vi "2086发送2.vi"() -> ()   [LabVIEW 2016, in "数据传输系统-06.lvlib"]
uses:
  <vilib>/Utility/config.llb/Write Key (String).vi
  <vilib>/Utility/config.llb/Read Key (String).vi
  <vilib>/Utility/config.llb/NI_LVConfig.lvlib
panel:
  out "数据发送起始时间":timestamp format="%<%.3X\n%Y/%m/%d>T"
  out "数据拆分":bool
  in  "设备类型":string(combo)="010200"
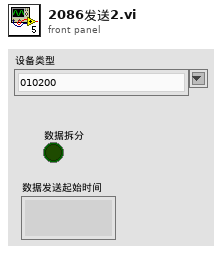
[diagram p1: front panel]
types:
  T1 = cluster{"CODMn":string, "CODCr":string, "DO":string, "铜":string, "PH":string, "氨氮":string, "比电导率":string, "水温":string, "COD":string, "浊度":string, "总氮":string, "总磷":string, "叶绿素a":string, "藻密度":string, "水位":string, "流速":string, "方向":string, "瞬时流量":string, "累积流量":string, "正累积流量":string, "负累积流量":string, "亚硝酸盐":string, "硫化物":string, "ORP":string, "铅":string, "镉":string, "锌":string, "镍":string, "锰":string, "汞":string, "气温":string, "气压":string, "风速":string, "风向":string, "空气温度":string, "相对湿度":string, "分钟雨量":string, "小时雨量":string, "日雨量":string, "累积雨量":string, "盐度":string, "磷酸盐":string, "硝氮":string, "氟化物":string, "挥发酚":string, "氯化物":string, "蓝绿藻":string, "余氯":string, "综合生物毒性":string, "艏向":string, "横摇":string, "纵摇":string, "分层标志":string, "层状态1":string, "层状态2":string, "水平平均流速":string, "流向":string, "北向流速分量":string, "东向流速分量":string, "垂直流速分量":string, "最大波高":string, "最大波周期":string, "1/10波高":string, "1/10波周期":string, "有效波高":string, "有效波周期":string, "平均波高":string, "平均波周期":string, "波向":string, "波个数":string, "水深":string, "X轴流速":string, "Y轴流速":string, "信号强度":string, "电压":string, "悬浮物":string}
  T2 = cluster{"QN":string, "ST":string, "CN":string, "PW":string, "MN":string, "FLAG":string, "PNUM":string, "PNO":string, "CP":string}
  T3 = typedef "LVComboBoxStrsAndValuesArrayTypeDef.ctl" = cluster{"String":string, "Value":string}[]
  T4 = typedef "数据传输系统-06.lvlib/应用环境.ctl" = enum16{"STD", "GB212", "婉仪平台"}
  T5 = cluster{"setini":string, "sysini":string, "hechaini":string, "actualwrite":string, "actualread":string, "datasent":string, "反控命令信息队列":string, "反控与仪器交互":string}
  T6 = cluster{"time1":string, "time2":string, "time3":string, "time4":string, "time5":string, "time6":string, "time7":string, "time8":string, "time9":string, "time10":string, "time11":string, "time12":string, "time13":string, "time14":string, "time15":string, "time16":string, "time17":string, "time18":string, "time19":string, "time20":string, "time21":string, "time22":string, "time23":string, "time24":string, "time25":string, "time26":string, "time27":string, "time28":string, "time29":string, "time30":string, "time31":string, "time32":string, "time33":string, "time34":string, "time35":string, "time36":string, "time37":string, "time38":string, "time39":string, "time40":string, "time41":string, "time42":string, "time43":string, "time44":string, "time45":string, "time46":string, "time47":string, "time48":string, "time49":string, "time50":string, "time51":string, "time52":string, "time53":string, "time54":string, "time55":string, "time56":string, "time57":string, "time58":string, "time59":string, "time60":string, "time61":string, "time62":string, "time63":string, "time64":string, "time65":string, "time66":string, "time67":string, "time68":string, "time69":string, "time70":string, "time71":string, "time72":string, "time73":string, "time74":string, "time75":string, "time76":string}
  T7 = cluster{"水样数据索引[0]":string, "水样数据索引[1]":string, "水样数据索引[2]":string, "水样数据索引[3]":string, "水样数据索引[4]":string, "水样数据索引[5]":string, "水样数据索引[6]":string, "水样数据索引[7]":string, "水样数据索引[8]":string, "水样数据索引[9]":string, "水样数据索引[10]":string, "水样数据索引[11]":string, "水样数据索引[12]":string, "水样数据索引[13]":string, "水样数据索引[14]":string, "水样数据索引[15]":string, "水样数据索引[16]":string, "水样数据索引[17]":string, "水样数据索引[18]":string, "水样数据索引[19]":string, "水样数据索引[20]":string, "水样数据索引[21]":string, "水样数据索引[22]":string, "水样数据索引[23]":string, "水样数据索引[24]":string, "水样数据索引[25]":string, "水样数据索引[26]":string, "水样数据索引[27]":string, "水样数据索引[28]":string, "水样数据索引[29]":string, "水样数据索引[30]":string, "水样数据索引[31]":string, "水样数据索引[32]":string, "水样数据索引[33]":string, "水样数据索引[34]":string, "水样数据索引[35]":string, "水样数据索引[36]":string, "水样数据索引[37]":string, "水样数据索引[38]":string, "水样数据索引[39]":string, "水样数据索引[40]":string, "水样数据索引[41]":string, "水样数据索引[42]":string, "水样数据索引[43]":string, "水样数据索引[44]":string, "水样数据索引[45]":string, "水样数据索引[46]":string, "水样数据索引[47]":string, "水样数据索引[48]":string, "水样数据索引[49]":string, "水样数据索引[50]":string, "水样数据索引[51]":string, "水样数据索引[52]":string, "水样数据索引[53]":string, "水样数据索引[54]":string, "水样数据索引[55]":string, "水样数据索引[56]":string, "水样数据索引[57]":string, "水样数据索引[58]":string, "水样数据索引[59]":string, "水样数据索引[60]":string, "水样数据索引[61]":string, "水样数据索引[62]":string, "水样数据索引[63]":string, "水样数据索引[64]":string, "水样数据索引[65]":string, "水样数据索引[66]":string, "水样数据索引[67]":string, "水样数据索引[68]":string, "水样数据索引[69]":string, "水样数据索引[70]":string, "水样数据索引[71]":string, "水样数据索引[72]":string, "水样数据索引[73]":string, "水样数据索引[74]":string, "水样数据索引[75]":string}
  T8 = typedef "NI_LVConfig.lvlib/Config Data RefNum.ctl" = refnum<k1>
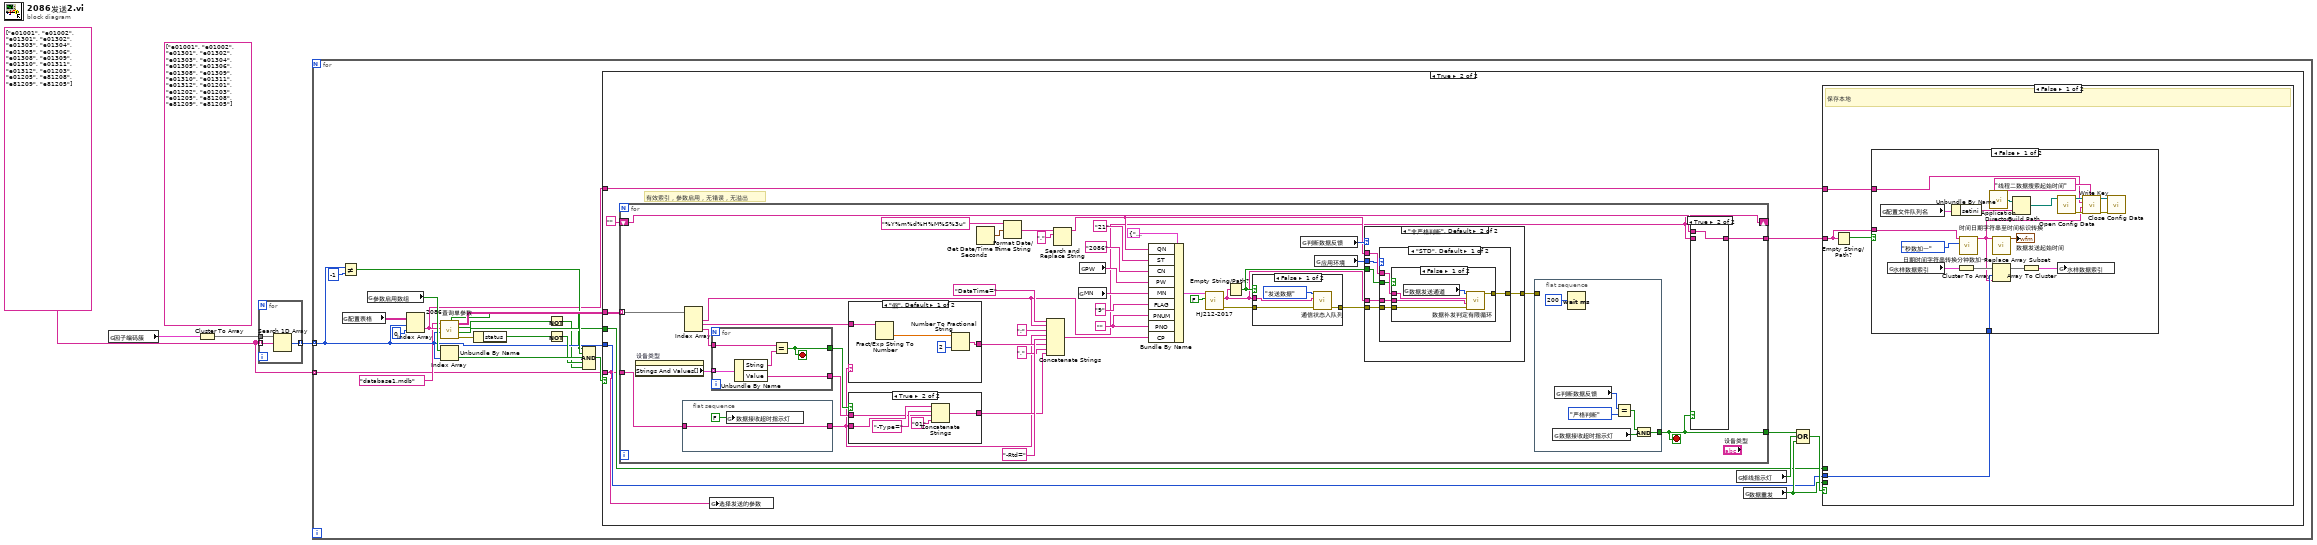
[diagram p0: block diagram]
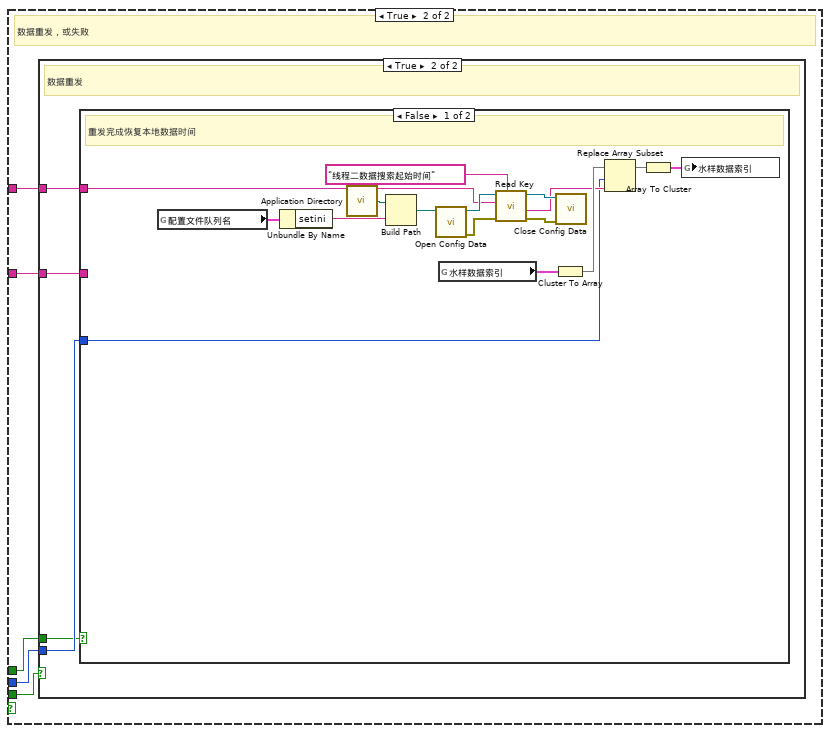
[diagram p4: hidden frame]
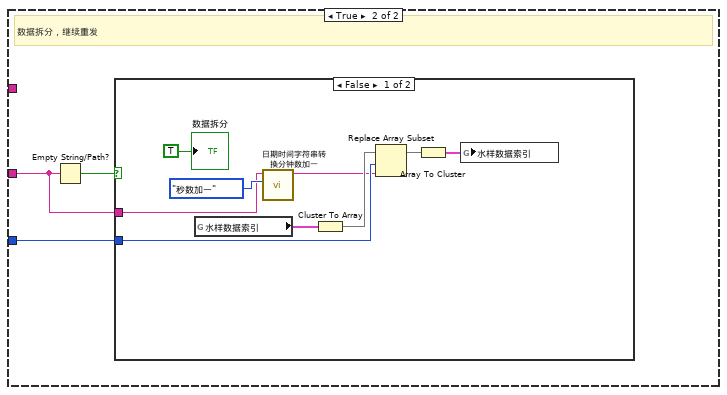
[diagram p6: hidden frame]
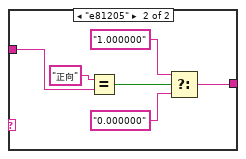
[diagram p9: hidden frame]
diagram:
  w1 = string[] ["e01001", "e01002", "e01301", "e01302", "e01303", "e01304", "e01305", "e01306", "e01308", "e01309", "e01310", "e01311", "e01312", "e01203", "e01205", "e81208", "e81209", "e81205"]
  (unwired) string[] ["e01001", "e01002", "e01301", "e01302", "e01303", "e01304", "e01305", "e01306", "e01308", "e01309", "e01310", "e01311", "e01312", "e01201", "e01202", "e01203", "e01205", "e81208", "e81209", "e81205"]
  n1 = global read "断电保存全局.vi" "因子编码簇"() -> (w4:T1)
  n2 = Cluster To Array(cluster=w4) -> (array=w3:string[])
  n3 = for {
    tunnel: w3 -> [w7]
    tunnel: w1 -> [w6] mode=indexing
    tunnel: [w5] -> w2 mode=indexing
    n4 = Search 1D Array(1D array=w7, element=w6) -> (index of element=w5:i32)  [unwired: 1 in]
  }
  n5 = for {
    tunnel: w2 -> [w11] mode=indexing
    tunnel: w1 -> [w10] mode=indexing
    n6 = Not Equal?(x=w11, y=-1) -> (x != y?=w21:bool)
    n7 = global read "断电保存全局.vi" "配置表格"() -> (w25:string[][])
    n8 = global read "断电保存全局.vi" "参数启用数组"() -> (w22:bool[])
    n9 = Index Array(array=w25, index (row)=w11, index (col)=0 ("y")) -> (element=w19:string)
    n10 = call "2086查询单参数.vi"("索引"=w11, "table"=w19, "database"="database1.mdb") -> ("error out"=w16:errorcluster, "拆分数据"=w17:bool, "database溢出"=w12:bool, "data"=w23:string[][], "有数据"=w8:bool)  [unwired: 4 in]
    n11 = Index Array(array=w22, index=w11) -> (element=w20:bool)
    n12 = Unbundle By Name(w16) -> ("status"=w15:bool)
    n13 = Not(x=w12) -> (.not. x?=w9:bool)
    n14 = Not(x=w15) -> (.not. x?=w14:bool)
    n15 = Compound Arithmetic op=AND ("复合运算")(w8, w21, w20, w14, w9) -> (w13:bool)
    n16 = case shown="True" w13 {
      tunnel: w23 -> [_ w37]
      tunnel: w10 -> [_ w27]
      tunnel: w19 -> [_ w32]
      tunnel: w11 -> [_ w31]
      tunnel: w17 -> [_ w30]
      frame False {
      }
      frame True {
        # "有效索引，参数启用，无错误，无溢出"
        n17 = for {
          tunnel: w37 -> [w106] mode=indexing
          tunnel: w27 -> [w98]
          tunnel: [w103] -> w36
          shift-right: [w101] -> _
          shift-left: "" -> [w102]
          tunnel: [w100] -> w29
          stop <- w103 stop-if-true
          w127 = ""
          n18 = property on="设备类型" class="CmbBox"() -> ("Strings And Values[]"=w120:T3)  [unwired: 2 in, 2 out]
          n19 = flat-sequence {
            tunnel: [w139] -> w99
            tunnel: w98 -> [w139]
            frame #0 {
              n20 = global write "全局 数据发送重叠.vi" "数据接收超时指示灯"(FALSE ("数据接收超时指示灯")) -> ()
            }
          }
          n21 = Index Array(array=w106) -> (element #1=w101:string, element #2=w105:string, element #3=w117:string)  [unwired: 3 in]
          n22 = for {
            tunnel: w120 -> [w188] mode=indexing
            tunnel: w117 -> [w186]
            tunnel: [w185] -> w118
            tunnel: [w184] -> w119
            stop <- w184 stop-if-true
            n23 = Unbundle By Name(w188) -> ("String"=w187:string, "Value"=w185:string)
            n24 = Equal?(x=w186, y=w187) -> (x = y?=w184:bool)
          }
          n25 = case shown="\"假\", Default" w99 {
            tunnel: w105 -> [w143 w151]
            tunnel: [w142 w146] -> w104
            frame "假", Default {
              n26 = Fract/Exp String To Number(string=w143) -> (number=w145:dbl)  [unwired: 3 in, 1 out]
              n27 = Number To Fractional String(number=w145, precision (6)=i16 2 ("精度(6)")) -> (F-format string=w142:string)  [unwired: 2 in]
            }
            frame "e81205" {
              n28 = Equal?(x="正向", y=w151) -> (x = y?=w149:bool)
              n29 = Select(t="1.000000" ("x"), s=w149, f="0.000000" ("x")) -> (s? t:f=w146:string)
            }
          }
          n30 = case shown="True" w119 {
            tunnel: w118 -> [_ w181]
            tunnel: w99 -> [_ w183]
            tunnel: [_ w179] -> w115
            frame False {
            }
            frame True {
              n31 = Concatenate Strings(w183, "-Type=" ("格式字符串"), w181, "01" ("字符串")) -> (w179:string)
            }
          }
          n32 = Get Date/Time In Seconds() -> (seconds since 1Jan1904=w135:timestamp)
          n33 = Format Date/Time String(time format string (%c)="%Y%m%d%H%M%S%3u" ("时间格式字符串(%c)"), seconds (now)=w135) -> (date/time string=w134:string)  [unwired: 1 in]
          n34 = Concatenate Strings("DataTime=" ("时间格式字符串(%c)"), w101, ";" ("字符串"), w99, "-Rtd=" ("时间格式字符串(%c)"), w104, "," ("字符串"), w115) -> (w125:string)
          n35 = Search and Replace String(input string=w134, search string="." ("搜索字符串")) -> (result string=w108:string)  [unwired: 6 in, 3 out]
          n36 = global read "断电保存全局.vi" "MN"() -> (w132:string)
          n37 = global read "断电保存全局.vi" "PW"() -> (w131:string)
          n38 = Bundle By Name(cluster=T2 {"QN"="", "ST"="", "CN"="", "PW"="", "MN"="", "FLAG"="", "PNUM"="", "PNO"="", "CP"=""} ("数据块"), "QN"=w108, "ST"="21", "CN"="2086", "PW"=w131, "MN"=w132, "FLAG"="9", "PNUM"=w127, "PNO"=w127, "CP"=w125) -> (w121:T2)
          n39 = call "HJ212-2017.vi"("PWD？"=FALSE, "数据段"=w121) -> ("error out"=w109:errorcluster, "通讯包字符串"=w110:string)  [unwired: 7 in, 1 out]
          n40 = Empty String/Path?(string/path=w110) -> (empty?=w114:bool)
          n41 = case shown="False" w114 {
            tunnel: [w161 w162] -> w112
            tunnel: w109 -> [w160 w162]
            tunnel: w110 -> [w158 _]
            frame False {
              n42 = call "通信状态入队列.vi"("错误输入（无错误）"=w160, "发送报文"=w158, "枚举"=enum16{"打开连接", "发送数据", "读取数据", "数据处理", "关闭连接"}."发送数据") -> ("错误输出"=w161:errorcluster)  [unwired: 8 in]
            }
            frame True {
            }
          }
          n43 = global read "断电保存全局.vi" "判断数据反馈"() -> (w111:enum16{"非严格判断", "严格判断", "不判断"})
          n44 = global read "断电保存全局.vi" "应用环境"() -> (w113:T4)
          n45 = case shown="\"非严格判断\", Default" w111 {
            tunnel: w110 -> [_ w168]
            tunnel: w112 -> [_ w167]
            tunnel: w108 -> [_ w166]
            tunnel: w113 -> [_ w165]
            tunnel: w114 -> [_ w164]
            tunnel: [_ w163] -> w107
            frame "不判断" {
            }
            frame "非严格判断", Default {
              n46 = case shown="\"STD\", Default" w165 {
                tunnel: w168 -> [w171 _]
                tunnel: w167 -> [w173 _]
                tunnel: w166 -> [w172 _]
                tunnel: w164 -> [w170 _]
                tunnel: [w169 _] -> w163
                frame "STD", Default {
                  n47 = case shown="False" w170 {
                    tunnel: w173 -> [w178 _]
                    tunnel: w172 -> [w176 _]
                    tunnel: w171 -> [w175 _]
                    tunnel: [w174 _] -> w169
                    frame False {
                      n48 = global read "断电保存全局.vi" "数据发送通道"() -> (w177:enum16{"TCP", "VISA"})
                      n49 = call "数据补发判定有限循环.vi"("错误输入（无错误）"=w178, "数据输入"=w175, "QN"=w176, "数据发送通道"=w177) -> ("error out"=w174:errorcluster)  [unwired: 7 in]
                    }
                    frame True {
                    }
                  }
                }
                frame "GB212" {
                }
              }
            }
          }
          n50 = flat-sequence {
            tunnel: w107 -> [_]
            tunnel: [w154] -> w103
            frame #0 {
              n51 = global read "全局 数据发送重叠.vi" "数据接收超时指示灯"() -> (w157:bool)
              n52 = global read "断电保存全局.vi" "判断数据反馈"() -> (w155:enum16{"非严格判断", "严格判断", "不判断"})
              n53 = Wait (ms)(milliseconds to wait=u32 200 ("等待时间（毫秒）")) -> ()  [unwired: 1 out]
              n54 = Equal?(x=w155, y=enum16{"非严格判断", "严格判断", "不判断"}."严格判断") -> (x = y?=w152:bool)
              n55 = And(x=w152, y=w157) -> (x .and. y?=w154:bool)
            }
          }
          n56 = case shown="True" w103 {
            tunnel: w102 -> [_ w141]
            tunnel: [w140 w141] -> w100
            tunnel: w101 -> [w140 _]
            frame False {
            }
            frame True {
            }
          }
        }
        n57 = global write "全局 水样时间.vi" "选择发送的参数"(w27) -> ()
        n58 = global read "全局 数据发送重叠.vi" "掉线指示灯"() -> (w35:bool)
        n59 = global read "断电保存全局.vi" "数据重发"() -> (w33:bool)
        n60 = Compound Arithmetic op=OR ("复合运算")(w36, w35, w33) -> (w34:bool)
        n61 = case shown="False" w34 {
          tunnel: w29 -> [w38 w61]
          tunnel: w31 -> [w40 w63]
          tunnel: w32 -> [w41 w65]
          tunnel: w33 -> [_ w64]
          tunnel: w30 -> [_ w62]
          frame False {
            # "保存本地"
            n62 = Empty String/Path?(string/path=w38) -> (empty?=w39:bool)
            n63 = case shown="False" w39 {
              tunnel: w41 -> [w53 _]
              tunnel: w40 -> [w47 _]
              tunnel: w38 -> [w42 _]
              frame False {
                n64 = global read "全局1.vi" "配置文件队列名"() -> (w43:T5)
                n65 = global read "全局 水样时间.vi" "水样数据索引"() -> (w48:T6)
                n66 = Unbundle By Name(w43) -> ("setini"=w44:string)
                n67 = Cluster To Array(cluster=w48) -> (array=w49:string[])
                n68 = call "日期时间字符串转换分钟数加一.vi"("枚举"=enum16{"分钟数加一", "秒数加一", "小时数加一"}."秒数加一", "data[0]"=w42) -> ("日期/时间字符串"=w46:string)  [unwired: 9 in]
                n69 = call <vilib>:"Application Directory.vi"() -> ("Application Directory"=w54:path)
                n70 = call "时间日期字符串至时间标识转换.vi"("时间日期字符串"=w46) -> ("时间标识"=→"数据发送起始时间":timestamp)  [unwired: 10 in]
                n71 = Replace Array Subset(array=w49, new element=w46, index=w47) -> (w50:string[])
                n72 = Build Path(base path=w54, name or relative path=w44) -> (appended path=w55:path)
                n73 = Array To Cluster(array=w50) -> (cluster=w51:T7)
                n74 = call <vilib>:"Open Config Data.vi"("configuration file path"=w55) -> ("error out"=w57:errorcluster, "refnum"=w56:T8)  [unwired: 8 in, 1 out]
                n75 = global write "全局 水样时间.vi" "水样数据索引"(w51) -> ()
                n76 = call-poly <vilib>:"Write Key.vi"("section"="线程二数据搜索起始时间", "error in (no error)"=w57, "value"=w46, "key"=w53, "refnum"=w56) -> ("error out"=w59:errorcluster, "refnum out"=w58:T8)  [unwired: 4 in, 1 out]
                n77 = call <vilib>:"Close Config Data.vi"("error in (no error)"=w59, "refnum"=w58) -> ()  [unwired: 8 in, 2 out]
              }
              frame True {
              }
            }
          }
          frame True {
            # "数据重发，或失败"
            n78 = case shown="True" w64 {
              tunnel: w65 -> [_ w69]
              tunnel: w63 -> [_ w68]
              tunnel: w62 -> [_ w67]
              tunnel: w61 -> [_ w66]
              frame False {
                # "数据发送失败"
              }
              frame True {
                # "数据重发"
                n79 = case shown="False" w67 {
                  tunnel: w69 -> [w73 _]
                  tunnel: w68 -> [w71 w88]
                  tunnel: w66 -> [_ w86]
                  frame False {
                    # "重发完成恢复本地数据时间"
                    n80 = global read "全局1.vi" "配置文件队列名"() -> (w70:T5)
                    n81 = Unbundle By Name(w70) -> ("setini"=w80:string)
                    n82 = call <vilib>:"Application Directory.vi"() -> ("Application Directory"=w74:path)
                    n83 = Build Path(base path=w74, name or relative path=w80) -> (appended path=w75:path)
                    n84 = call <vilib>:"Open Config Data.vi"("configuration file path"=w75) -> ("error out"=w81:errorcluster, "refnum"=w76:T8)  [unwired: 8 in, 1 out]
                    n85 = global read "全局 水样时间.vi" "水样数据索引"() -> (w82:T6)
                    n86 = call-poly <vilib>:"Read Key.vi"("section"="线程二数据搜索起始时间", "error in (no error)"=w81, "key"=w73, "refnum"=w76) -> ("error out"=w79:errorcluster, "value"=w72:string, "refnum out"=w78:T8)  [unwired: 4 in, 1 out]
                    n87 = Cluster To Array(cluster=w82) -> (array=w83:string[])
                    n88 = call <vilib>:"Close Config Data.vi"("error in (no error)"=w79, "refnum"=w78) -> ()  [unwired: 8 in, 2 out]
                    n89 = Replace Array Subset(array=w83, new element=w72, index=w71) -> (w84:string[])
                    n90 = Array To Cluster(array=w84) -> (cluster=w85:T7)
                    n91 = global write "全局 水样时间.vi" "水样数据索引"(w85) -> ()
                  }
                  frame True {
                    # "数据拆分，继续重发"
                    n92 = Empty String/Path?(string/path=w86) -> (empty?=w87:bool)
                    n93 = case shown="False" w87 {
                      tunnel: w88 -> [w92 _]
                      tunnel: w86 -> [w89 _]
                      frame False {
                        n94 = global read "全局 水样时间.vi" "水样数据索引"() -> (w93:T6)
                        n95 = call "日期时间字符串转换分钟数加一.vi"("枚举"=enum16{"分钟数加一", "秒数加一", "小时数加一"}."秒数加一", "data[0]"=w89) -> ("日期/时间字符串"=w91:string)  [unwired: 9 in]
                        n96 = Cluster To Array(cluster=w93) -> (array=w94:string[])
                        n97 = Replace Array Subset(array=w94, new element=w91, index=w92) -> (w95:string[])
                        n98 = Array To Cluster(array=w95) -> (cluster=w96:T7)
                        n99 = global write "全局 水样时间.vi" "水样数据索引"(w96) -> ()
                        "数据拆分" <- TRUE
                      }
                      frame True {
                      }
                    }
                  }
                }
              }
            }
          }
        }
      }
    }
  }
